vi "Get Image Subset.vi"(7 "Image Units":T2, 8 "error in (no error)":errorcluster, 10 "Rectangle":T1, 11 "Image":T3) -> (0 "error out":errorcluster, 3 "Image Subset":T3)   [LabVIEW 2020, in "MacroAssert.lvlib" / "Image Assertion.lvclass"]
uses:
  Image Assertion.lvclass
  Image Assertion.lvclass/Image Assertion.ctl
  <vilib>/picture/picture.llb/imagedata.ctl
  Image Units.ctl
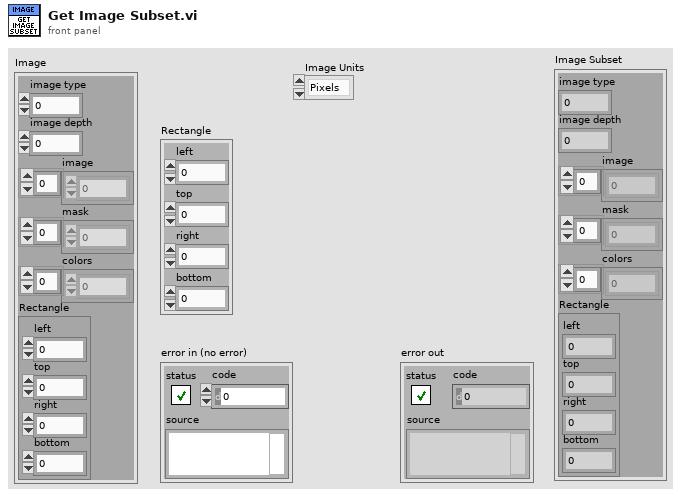
[diagram p1: front panel]
types:
  T1 = cluster{"left":i16, "top":i16, "right":i16, "bottom":i16}
  T2 = typedef "MacroAssert.lvlib/Image Assertion.lvclass/Image Units.ctl" = enum16{"Pixels", "Percent"}
  T3 = typedef "imagedata.ctl" = cluster{"image type":i32, "image depth":i32, "image":u8[], "mask":u8[], "colors":u32[], "Rectangle":cluster{"left":i16, "top":i16, "right":i16, "bottom":i16}}
  T4 = cluster{"left":dbl, "top":dbl, "right":dbl, "bottom":dbl}
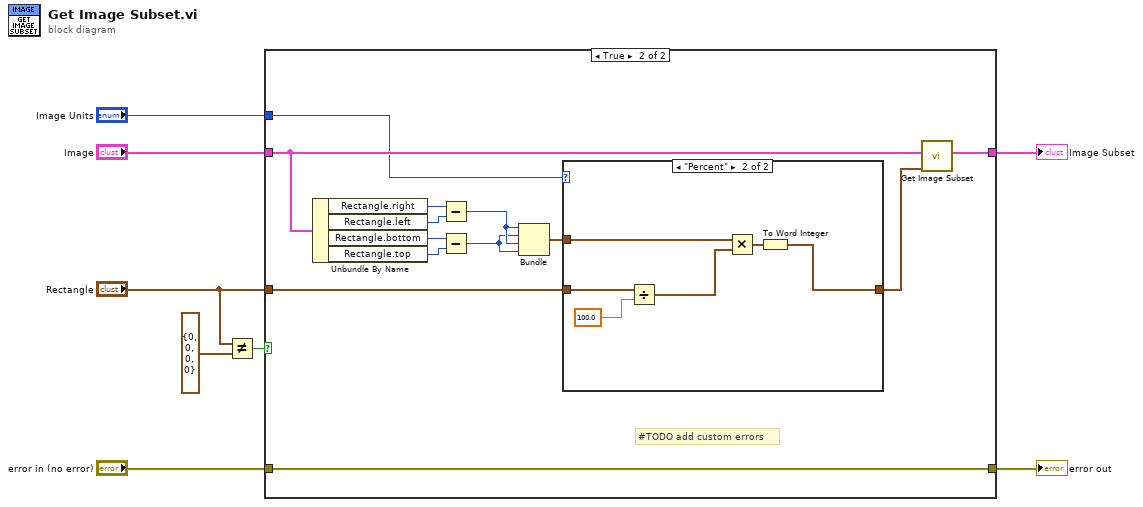
[diagram p0: block diagram]
diagram:
  n1 = Not Equal?(x="Rectangle", y=T1 {"left"=0, "top"=0, "right"=0, "bottom"=0}) -> (x != y?=w5:bool)
  n2 = case shown="True" w5 {
    tunnel: [w10 w23] -> w8
    tunnel: "Image" -> [w10 w22]
    tunnel: "Image Units" -> [_ w20]
    tunnel: "error in (no error)" -> [w9 w11]
    tunnel: "Rectangle" -> [_ w21]
    tunnel: [w9 w11] -> w1
    frame False {
    }
    frame True {
      # "#TODO add custom errors"
      n3 = Unbundle By Name(w22) -> ("Rectangle.right"=w18:i16, "Rectangle.left"=w17:i16, "Rectangle.bottom"=w16:i16, "Rectangle.top"=w15:i16)
      n4 = Subtract(x=w18, y=w17) -> (x-y=w13:i16)
      n5 = Subtract(x=w16, y=w15) -> (x-y=w12:i16)
      n6 = Bundle(w13, w12, w13, w12) -> (w14:cluster{i16, i16, i16, i16})  [unwired: 1 in]
      n7 = case shown="\"Percent\"" w20 {
        tunnel: w21 -> [w24 w30]
        tunnel: [w24 w25] -> w19
        tunnel: w14 -> [_ w28]
        frame "Pixels" {
        }
        frame "Percent" {
          n8 = Divide(x=w30, y=100.0) -> (x/y=w27:T4)
          n9 = Multiply(x=w28, y=w27) -> (x*y=w26:cluster{dbl, dbl, dbl, dbl})
          n10 = To Word Integer(number=w26) -> (16bit integer=w25:cluster{i16, i16, i16, i16})
        }
      }
      n11 = call <vilib>:"Get Image Subset.vi"("subset rect"=w19, "image data"=w22) -> ("image subset"=w23:T3)  [unwired: 4 in, 1 out]
    }
  }
  "error out" <- w1
  "Image Subset" <- w8
